vi "Lift Init.vi"   [LabVIEW 2014]
uses:
  Begin/Global Variables.vi
  Begin/Global RefNums.vi
types:
  T1 = typedef "WPI_SwitchDevRef.ctl" = cluster{"DevStatus":errorcluster, "DIO Channel":T2, "Controller":T3, "CntIndex":T4, "Normally Closed":bool}
  T2 = typedef "FPGA_DIOChannel.ctl" = enum8{"DIO 0", "DIO 1", "DIO 2", "DIO 3", "DIO 4", "DIO 5", "DIO 6", "DIO 7", "DIO 8", "DIO 9", "DIO MXP 0", "DIO MXP 1", "DIO MXP 2", "DIO MXP 3", "DIO MXP 4", "DIO MXP 5", "DIO MXP 6", "DIO MXP 7", "DIO MXP 8", "DIO MXP 9", "DIO MXP 10", "DIO MXP 11", "DIO MXP 12", "DIO MXP 13", "DIO MXP 14", "DIO MXP 15", "Invalid"}
  T3 = typedef "FPGA_TypedefDigitalModule.ctl" = enum16{"Controller 1"}
  T4 = typedef "FPGA_CounterCtrSystemIndex.ctl" = enum8{"Ctr 0", "Ctr 1", "Ctr 2", "Ctr 3", "Ctr 4", "Ctr 5", "Ctr 6", "Ctr 7", "Invalid"}
  T5 = typedef "WPI_EncoderDevRef.ctl" = cluster{"DevStatus":errorcluster, "EncoderIndex":T6, "CounterIndex":T4, "DistancePerCount":dbl, "Decoding Type":T7}
  T6 = typedef "FPGA_EncoderIdx.ctl" = enum8{"Enc 0", "Enc 1", "Enc 2", "Enc 3", "Enc 4", "Enc 5", "Enc 6", "Enc 7", "Invalid"}
  T7 = typedef "WPI_EncoderType.ctl" = enum16{"1x", "2x", "4x"}
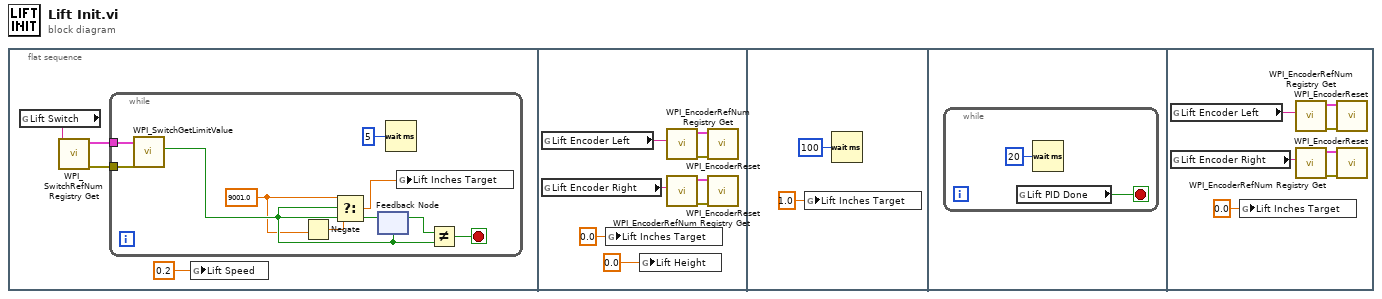
[diagram p0: block diagram]
diagram:
  n1 = flat-sequence {
    frame #0 {
      n2 = global read "Global RefNums.vi" "Lift Switch"() -> (w1:string)
      n3 = call <vilib>:"WPI_SwitchRefNum Registry Get.vi"("refnum name"=w1) -> ("error out"=w2:errorcluster, "SwitchDevRef"=w3:T1)  [unwired: 9 in]
      n4 = while {
        tunnel: w3 -> [w10]
        tunnel: w2 -> [w9]
        stop <- w12 stop-if-true
        w6 = 9001.0 ("y")
        n5 = call <vilib>:"WPI_SwitchGetLimitValue.vi"("error in (no error)"=w9, "SwitchDevRef"=w10) -> ("Switch Pressed"=w8:bool)  [unwired: 7 in, 2 out]
        n6 = Negate(x=w6) -> (-x=w7:dbl)
        n7 = Select(t=w6, s=w8, f=w7) -> (s? t:f=w5:dbl)
        n8 = feedback-in #1(w8) -> ()
        n9 = feedback #1(w8) -> (w13:bool)
        n10 = Wait (ms)(milliseconds to wait=u32 5) -> ()  [unwired: 1 out]
        n11 = global write "Global Variables.vi" "Lift Inches Target"(w5) -> ()
        n12 = Not Equal?(x=w13, y=w8) -> (x != y?=w12:bool)
      }
      n13 = global write "Global Variables.vi" "Lift Speed"(0.2 ("t")) -> ()
    }
    frame #1 {
      n14 = global read "Global RefNums.vi" "Lift Encoder Left"() -> (w18:string)
      n15 = global read "Global RefNums.vi" "Lift Encoder Right"() -> (w17:string)
      n16 = global write "Global Variables.vi" "Lift Inches Target"(0.0 ("Lift Inches Target")) -> ()
      n17 = global write "Global Variables.vi" "Lift Height"(0.0 ("Lift Inches Target")) -> ()
      n18 = call <vilib>:"WPI_EncoderRefNum Registry Get.vi"("refnum name"=w18) -> ("error out"=w21:errorcluster, "EncoderDevRef"=w16:T5)  [unwired: 9 in]
      n19 = call <vilib>:"WPI_EncoderRefNum Registry Get.vi"("refnum name"=w17) -> ("error out"=w19:errorcluster, "EncoderDevRef"=w20:T5)  [unwired: 9 in]
      n20 = call <vilib>:"WPI_EncoderReset.vi"("error in (no error)"=w21, "EncoderDevRef"=w16) -> ()  [unwired: 8 in, 2 out]
      n21 = call <vilib>:"WPI_EncoderReset.vi"("error in (no error)"=w19, "EncoderDevRef"=w20) -> ()  [unwired: 8 in, 2 out]
    }
    frame #2 {
      n22 = global write "Global Variables.vi" "Lift Inches Target"(1.0 ("Lift Inches Target")) -> ()
      n23 = Wait (ms)(milliseconds to wait=u32 100) -> ()  [unwired: 1 out]
    }
    frame #3 {
      n24 = while {
        stop <- w24 stop-if-true
        n25 = global read "Global Variables.vi" "Lift PID Done"() -> (w24:bool)
        n26 = Wait (ms)(milliseconds to wait=u32 20) -> ()  [unwired: 1 out]
      }
    }
    frame #4 {
      n27 = global read "Global RefNums.vi" "Lift Encoder Left"() -> (w31:string)
      n28 = global read "Global RefNums.vi" "Lift Encoder Right"() -> (w32:string)
      n29 = global write "Global Variables.vi" "Lift Inches Target"(0.0 ("Lift Inches Target")) -> ()
      n30 = call <vilib>:"WPI_EncoderRefNum Registry Get.vi"("refnum name"=w31) -> ("error out"=w28:errorcluster, "EncoderDevRef"=w27:T5)  [unwired: 9 in]
      n31 = call <vilib>:"WPI_EncoderRefNum Registry Get.vi"("refnum name"=w32) -> ("error out"=w30:errorcluster, "EncoderDevRef"=w29:T5)  [unwired: 9 in]
      n32 = call <vilib>:"WPI_EncoderReset.vi"("error in (no error)"=w28, "EncoderDevRef"=w27) -> ()  [unwired: 8 in, 2 out]
      n33 = call <vilib>:"WPI_EncoderReset.vi"("error in (no error)"=w30, "EncoderDevRef"=w29) -> ()  [unwired: 8 in, 2 out]
    }
  }
